vi "sub_group_start-finish.vi"(7 "cmd":enum16{"Start", "Finish"}(ring), 8 "error in":errorcluster, 11 "count":i32) -> (0 "error out":errorcluster)   [LabVIEW 2019]
uses:
  _ctrl/rw.ctl
  SubVIs/common/_ctrl/system-status.ctl
  cmd_timecheck.ctl
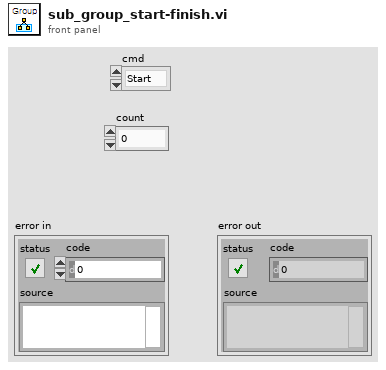
[diagram p1: front panel]
types:
  T1 = typedef "system-status.ctl" = enum16{"Initial", "Update", "Clear", "Read"}
  T2 = typedef "rw.ctl" = enum16{"read", "write"}
  T3 = typedef "cmd_timecheck.ctl" = enum16{"Group start", "Group end", "Grout dt", "Ch start", "Ch end", "Ch dt", "init", "NF start", "NF stop", "idrc start", "idrc stop", "scope start", "scope stop", "ao start", "ao stop", "relay start", "relay stop", "NF read start", "NF read stop", "NF set start", "NF set stop", "idrc level start", "idrc level stop", "scope trig start", "scope trig stop", "relay dischar star", "relay dischar stop", "data process start", "data process stop", "ch-relay on start", "ch-relay on stop", "hw set start", "hw set stop", "pwr-in on start", "pwr-in on stop", "pwr-out on start", "pwr-out on stop", "ao on start", "ao on stop", "ao 0v start", "ao 0v stop", "pwr-in off start", "pwr-in off stop", "relay-all off start", "relay-all off stop", "pwr-out off start", "pwr-out off stop", "discharge start", "discharge stop", "950 read start", "950 read stop"}
  T4 = typedef "Testing-info.ctl" = cluster{"전체채널수":u8, "현재채널번호":u8, "Irms":dbl, "입력전압":dbl, "입력전류":dbl, "출력전압":dbl, "출력전류":dbl, "온도":dbl, "제어단 단선":bool, "제어단 단락":bool, "제어단 특성변화":bool, "출력단 단선":bool, "출력단 단락":bool, "출력단 특성변화":bool, "출력단 전압":bool, "카운트 일치":bool, "Irms 판정":bool, "온도":bool, "테스트 회수":u32, "TestType":T5, "현재회수":u32, "Ch selection":cluster{"1ch":bool, "2ch":bool, "3ch":bool, "4ch":bool, "5ch":bool, "6ch":bool}, "반복":u32, "Path":path, "파일생성주기":u32, "start time":dbl, "stop time":dbl, "현재반복회수":u32, "NG":cluster{"입출력 카운트":bool, "출력전류RMS":bool}}
  T5 = typedef "sequence_single.ctl" = enum16{"Register", "RC", "B1", "B2", "B3", "Oper_LV", "Oper_HV", "ContR_LV"}
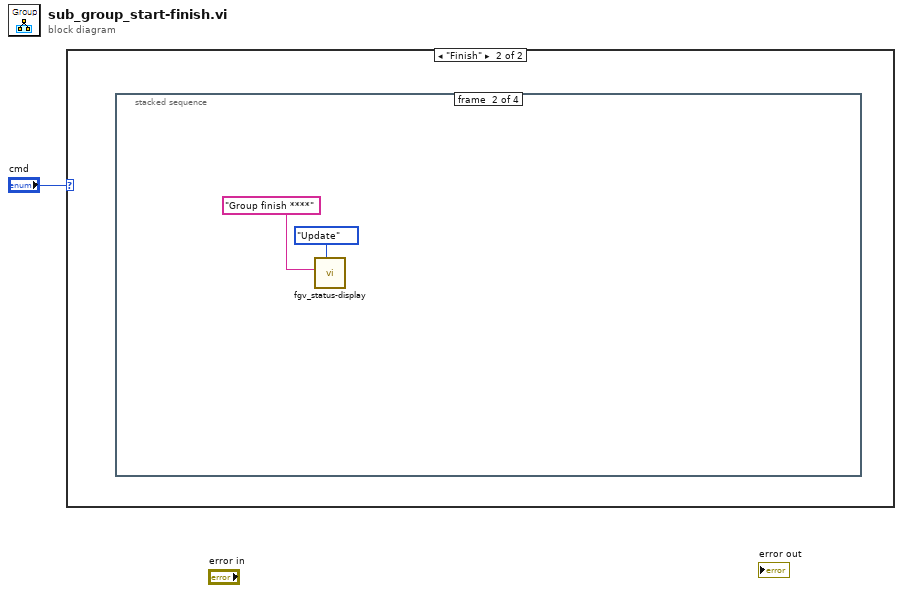
[diagram p0: block diagram]
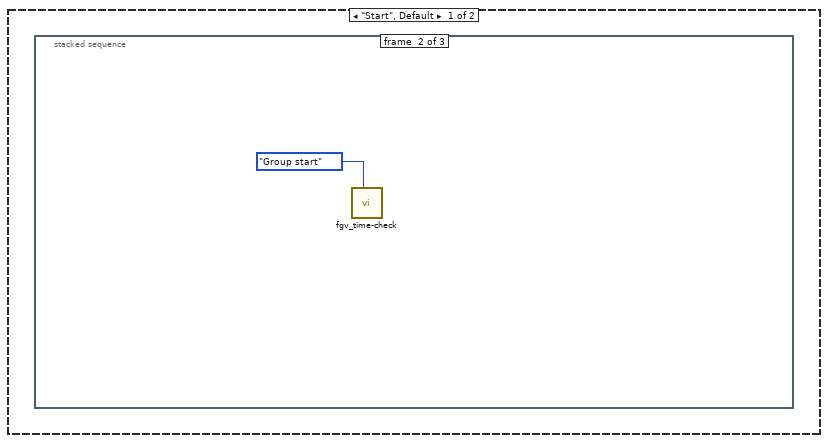
[diagram p2: hidden frame]
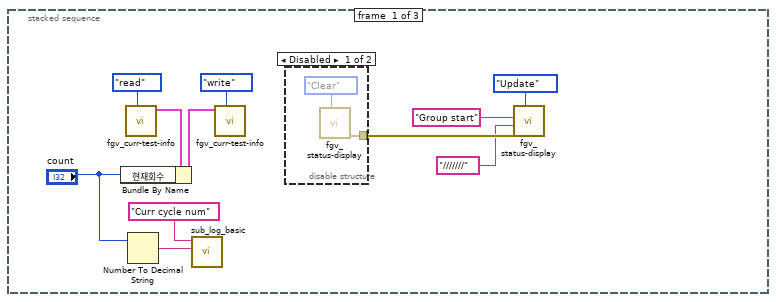
[diagram p3: hidden frame]
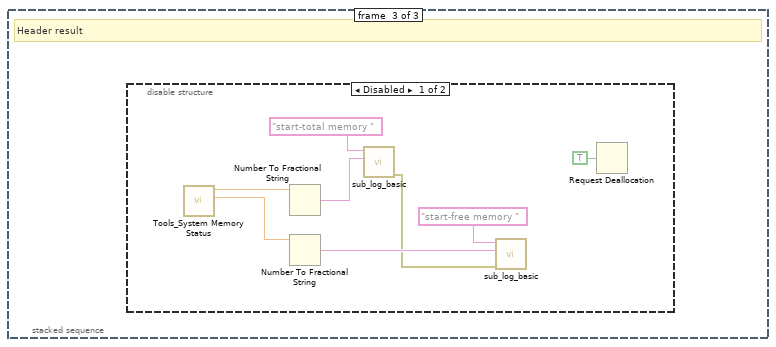
[diagram p5: hidden frame]
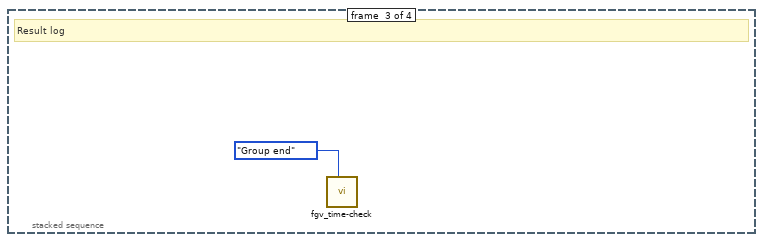
[diagram p8: hidden frame]
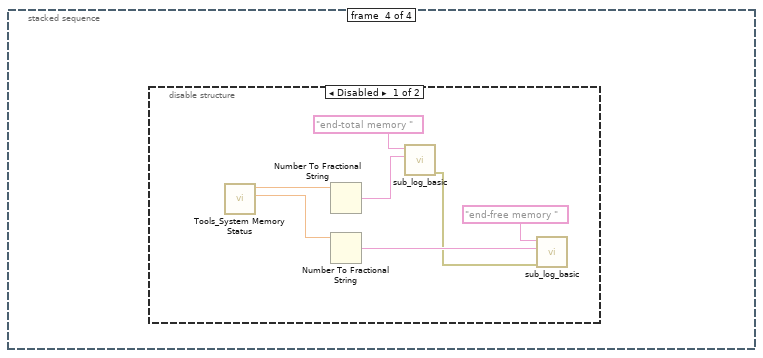
[diagram p9: hidden frame]
diagram:
  n1 = case shown="\"Finish\"" "cmd" {
    frame "Start", Default {
      n2 = stacked-sequence {
        frame #0 {
          n3 = call "fgv_curr-test-info.vi"("cmd"=rw."read") -> ("현재테스트 정보 2"=w11:T4)  [unwired: 10 in]
          n4 = Bundle By Name(cluster=w11, "현재회수"="count") -> (w12:T4)
          n5 = Number To Decimal String(number="count") -> (decimal integer string=w6:string)  [unwired: 1 in]
          n6 = call "sub_log_basic.vi"("desc"=w6, "Title"="Curr cycle num") -> ()  [unwired: 9 in, 1 out]
          n7 = call "fgv_curr-test-info.vi"("cmd"=rw."write", "현재테스트 정보"=w12) -> ()  [unwired: 9 in, 1 out]
          n8 = disable-structure shown="Disabled" {
            disable-tunnel: [w13 _] -> w4
            frame Disabled {
              n9 = call "fgv_status-display.vi"("Mode"=system-status."Clear") -> ("error out"=w13:errorcluster)  [unwired: 10 in]
            }
            frame Enabled {
            }
          }
          n10 = call "fgv_status-display.vi"("Mode"=system-status."Update", "error in"=w4, "detail"="///////" ("title"), "title"="Group start") -> ()  [unwired: 7 in, 1 out]
        }
        frame #1 {
          n11 = call "fgv_time-check.vi"("cmd"=cmd_timecheck."Group start") -> ()  [unwired: 9 in, 2 out]
        }
        frame #2 {
          # "Header result"
          n12 = disable-structure shown="Disabled" {
            frame Disabled {
              n13 = call "Tools_System Memory Status.vi"() -> ("Free memory (MB)"=w22:dbl, "Total memory (MB)"=w17:dbl)  [unwired: 8 in, 2 out]
              n14 = Number To Fractional String(number=w17) -> (F-format string=w18:string)  [unwired: 3 in]
              n15 = Number To Fractional String(number=w22) -> (F-format string=w21:string)  [unwired: 3 in]
              n16 = call "sub_log_basic.vi"("desc"=w18, "Title"="start-total memory ") -> ("error out"=w19:errorcluster)  [unwired: 9 in]
              n17 = call "sub_log_basic.vi"("error in"=w19, "desc"=w21, "Title"="start-free memory ") -> ()  [unwired: 8 in, 1 out]
              n18 = Request Deallocation(TRUE ("flag")) -> ()
            }
            frame Enabled {
            }
          }
        }
      }
    }
    frame "Finish" {
      n19 = stacked-sequence {
        frame #0 {
        }
        frame #1 {
          n20 = call "fgv_status-display.vi"("Mode"=system-status."Update", "title"="Group finish ****") -> ()  [unwired: 9 in, 1 out]
        }
        frame #2 {
          # "Result log"
          n21 = call "fgv_time-check.vi"("cmd"=cmd_timecheck."Group end") -> ()  [unwired: 9 in, 2 out]
        }
        frame #3 {
          n22 = disable-structure shown="Disabled" {
            frame Disabled {
              n23 = call "Tools_System Memory Status.vi"() -> ("Free memory (MB)"=w32:dbl, "Total memory (MB)"=w27:dbl)  [unwired: 8 in, 2 out]
              n24 = Number To Fractional String(number=w27) -> (F-format string=w28:string)  [unwired: 3 in]
              n25 = Number To Fractional String(number=w32) -> (F-format string=w31:string)  [unwired: 3 in]
              n26 = call "sub_log_basic.vi"("desc"=w28, "Title"="end-total memory ") -> ("error out"=w29:errorcluster)  [unwired: 9 in]
              n27 = call "sub_log_basic.vi"("error in"=w29, "desc"=w31, "Title"="end-free memory ") -> ()  [unwired: 8 in, 1 out]
            }
            frame Enabled {
            }
          }
        }
      }
    }
  }
